vi "oscRead.vi"(0 "input cluster":T2, 1 "error in":errorcluster caption="Error in" {"code" format="%.0x"}) -> (2 "appended array":T1(array[cluster]), 3 "Output String":string, 4 "error out (no error)":errorcluster)   [LabVIEW 2011]
uses:
  Server_Globals.vi
  <instrlib>/niScope/Acquire/Fetch/niScope Multi Fetch Binary 8.vi
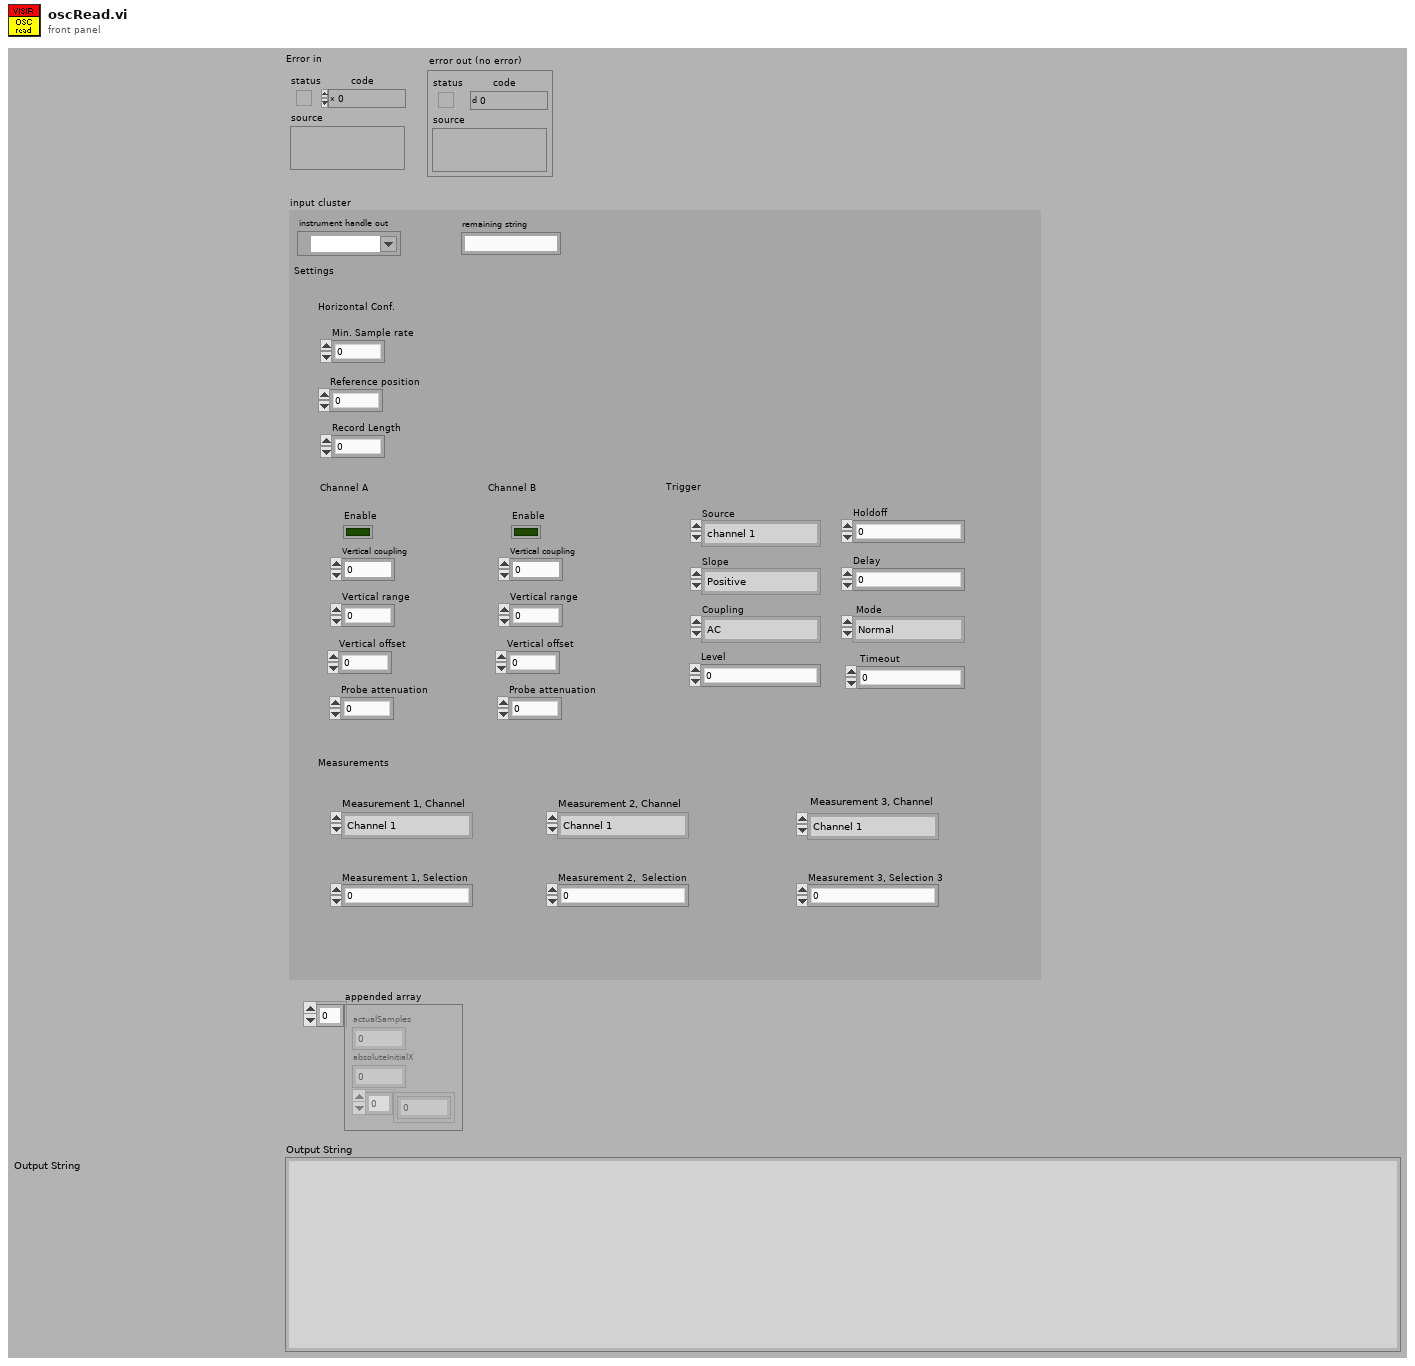
[diagram p1: front panel]
types:
  T1 = cluster{"actualSamples":i32, "absoluteInitialX":dbl, dbl[]}[]
  T2 = cluster{"instrument handle out":refnum<k15>, "remaining string":string, "Settings":cluster{"Horizontal Conf.":cluster{"Min. Sample rate":dbl, "Reference position":dbl, "Record Length":i16}, "Channel A":cluster{"Enable":bool, "Vertical coupling":dbl, "Vertical range":dbl, "Vertical offset":dbl, "Probe attenuation":dbl}, "Channel B":cluster{"Enable":bool, "Vertical coupling":dbl, "Vertical range":dbl, "Vertical offset":dbl, "Probe attenuation":dbl}, "Trigger":cluster{"Source":enum8{"channel 1", "channel 2", "Imediate", "External trigger"}, "Slope":enum8{"Positive", "Negative"}, "Coupling":enum8{"AC", "DC"}, "Level":dbl, "Holdoff":dbl, "Delay":dbl, " Timeout":dbl, " Mode":enum8{"Normal", "Auto", "Auto Level", ""}}, "Measurements":cluster{"Measurement 1, Channel":enum8{"Channel 1", "Channel 2", "Channel 3", "Channel 4"}, "Measurement 1, Selection":dbl, "Measurement 2, Channel":enum8{"Channel 1", "Channel 2", "Channel 3", "Channel 4"}, "Measurement 2,  Selection":dbl, "Measurement 3, Channel":enum8{"Channel 1", "Channel 2", "Channel 3", "Channel 4"}, "Measurement 3, Selection 3":dbl}}}
  T3 = cluster{"I/O Settings":u64[], "Instrument Handle":cluster{"5402":refnum<k15>, " 5112":refnum<k15>, "4072":refnum<k15>, "USB":refnum<visa-resource-name>, "4110":refnum<k15>}, "Logfile":refnum<file>, "Log Level":i8, "Clear":i32[], "OS Set":cluster{"instrument handle out":refnum<k15>, "remaining string":string, "Settings":cluster{"Horizontal Conf.":cluster{"Min. Sample rate":dbl, "Reference position":dbl, "Record Length":i16}, "Channel A":cluster{"Enable":bool, "Vertical coupling":dbl, "Vertical range":dbl, "Vertical offset":dbl, "Probe attenuation":dbl}, "Channel B":cluster{"Enable":bool, "Vertical coupling":dbl, "Vertical range":dbl, "Vertical offset":dbl, "Probe attenuation":dbl}, "Trigger":cluster{"Source":enum8{"channel 1", "channel 2", "Imediate", "External trigger"}, "Slope":enum8{"Positive", "Negative"}, "Coupling":enum8{"AC", "DC"}, "Level":dbl, "Holdoff":dbl, "Delay":dbl, " Timeout":dbl, " Mode":enum8{"Normal", "Auto", "Auto Level"}}, "Measurements":cluster{"Measurement 1, Channel":enum8{"Channel 1", "Channel 2", "Channel 3", "Channel 4"}, "Measurement 1, Selection":u16, "Measurement 2, Channel":enum8{"Channel 1", "Channel 2", "Channel 3", "Channel 4"}, "Measurement 2,  Selection":u16, "Measurement 3, Channel":enum8{"Channel 1", "Channel 2", "Channel 3", "Channel 4"}, "Measurement 3, Selection 3":u16}}}, "DC Power Supply":cluster{"0":refnum<k15>, "1":refnum<k15>, "2":refnum<k15>, "3":refnum<k15>, "4":refnum<k15>}, "USB Interface":cluster{"0":refnum<visa-resource-name>, "1":refnum<visa-resource-name>, "2":refnum<visa-resource-name>, "3":refnum<visa-resource-name>, "4":refnum<visa-resource-name>}, "Function Generator":cluster{"0":refnum<k15>, "1":refnum<k15>, "2":refnum<k15>, "3":refnum<k15>, "4":refnum<k15>}, "Digital Multimeter":cluster{"0":refnum<k15>, "1":refnum<k15>, "2":refnum<k15>, "3":refnum<k15>, "4":refnum<k15>}, "Digital Osciliscope":cluster{"0":refnum<k15>, "1":refnum<k15>, "2":refnum<k15>, "3":refnum<k15>, "4":refnum<k15>}, "To M Server":string, "Adres":string[][], "Matrix version":string, "MD5":string, "Digital Multimeter Card 2":cluster{"0":string, "1":string, "2":string, "3":string, "4":string}}
  T4 = cluster{"0":refnum<k15>, "1":refnum<k15>, "2":refnum<k15>, "3":refnum<k15>, "4":refnum<k15>}
  T5 = cluster{"Measurement 1, Channel":enum8{"Channel 1", "Channel 2", "Channel 3", "Channel 4"}, "Measurement 1, Selection":dbl, "Measurement 2, Channel":enum8{"Channel 1", "Channel 2", "Channel 3", "Channel 4"}, "Measurement 2,  Selection":dbl, "Measurement 3, Channel":enum8{"Channel 1", "Channel 2", "Channel 3", "Channel 4"}, "Measurement 3, Selection 3":dbl}
  T6 = cluster{"actualSamples":i32, "absoluteInitialX":dbl, "relativeInitialX":dbl, "xIncrement":dbl, "offset":dbl, "gain":dbl, "reserved1":dbl, "reserved2":dbl}[]
  T7 = cluster{"Vertical Coupling":i32, "Vertical Coupling":i32}
  T8 = cluster{cluster{"Enable":bool, "Enable":bool}, cluster{"Vertical Coupling":i32, "Vertical Coupling":i32}}
  T9 = cluster{" result ":dbl, " result  2":dbl, " result  3":dbl}
  T10 = cluster{"actualSamples":i32, "absoluteInitialX":dbl, "relativeInitialX":dbl, "xIncrement":dbl, "offset":dbl, "gain":dbl, "reserved1":dbl, "reserved2":dbl}
  T11 = cluster{"actualSamples":i32, "absoluteInitialX":dbl, dbl[]}
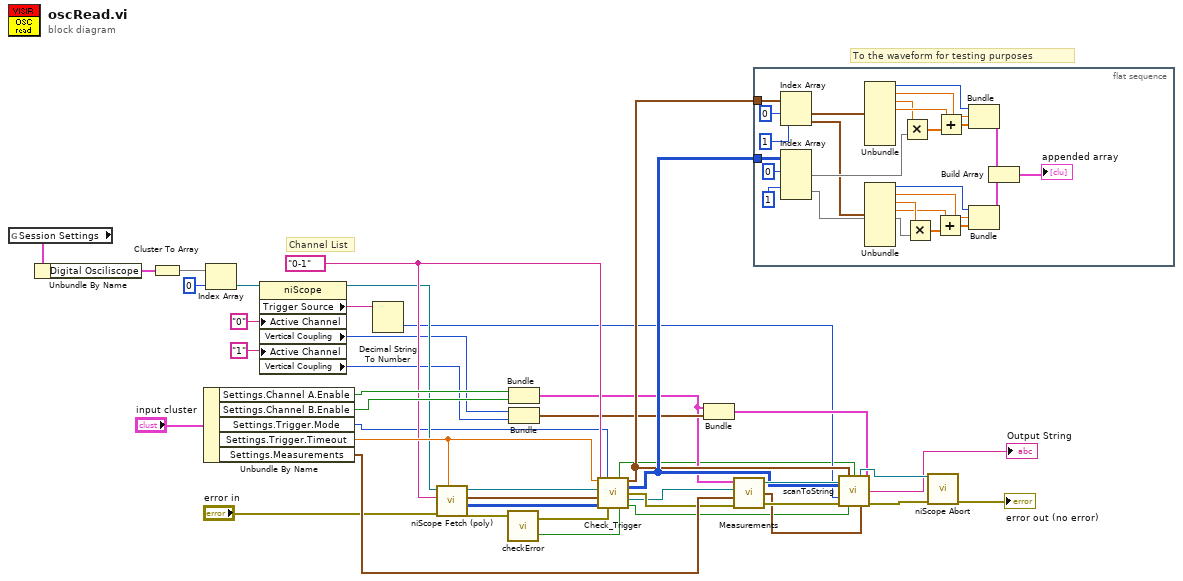
[diagram p0: block diagram]
diagram:
  w20 = "0-1" ("channelList")
  # "Channel List"
  # "To the waveform for testing purposes"
  n1 = global read "Server_Globals.vi" "Session Settings"() -> (w6:T3)
  n2 = Unbundle By Name(w6) -> ("Digital Osciliscope"=w5:T4)
  n3 = Cluster To Array(cluster=w5) -> (array=w4:refnum<k15>[])
  n4 = Unbundle By Name("input cluster") -> ("Settings.Channel A.Enable"=w22:bool, "Settings.Channel B.Enable"=w21:bool, "Settings.Trigger.Mode"=w9:enum8{"Normal", "Auto", "Auto Level", ""}, "Settings.Trigger.Timeout"=w31:dbl, "Settings.Measurements"=w35:T5)
  n5 = Index Array(array=w4, index=0) -> (element=w2:refnum<k15>)
  n6 = property class="niScope"(reference=w2, "Active Channel"="0", "Active Channel"="1") -> (reference out=w14:refnum<k15>, "Trigger Source"=w8:string, "Vertical Coupling"=w11:i32, "Vertical Coupling"=w10:i32)  [unwired: 1 in, 1 out]
  n7 = Decimal String To Number(string=w8) -> (number=w7:i32)  [unwired: 2 in, 1 out]
  n8 = call-poly <instrlib>:"niScope Fetch (poly).vi"("timeout"=w31, "error in"="error in", "channels"=w20, "instrument handle"=w14) -> ("error out"=w40:errorcluster, "wfm"=w29:i8[][], "wfm info"=w41:T6, "instrument handle out"=w30:refnum<k15>)  [unwired: 4 in]
  n9 = call "checkError.vi"("error in"=w40) -> ("Time out"=w33:bool, "error out"=w28:errorcluster)  [unwired: 1 in]
  n10 = Bundle("Enable"=w22, "Enable"=w21) -> (w18:cluster{"Enable":bool, "Enable":bool})  [unwired: 1 in]
  n11 = Bundle("Vertical Coupling"=w11, "Vertical Coupling"=w10) -> (w19:T7)  [unwired: 1 in]
  n12 = call "Check_Trigger.vi"("Timeout"=w31, "Mode"=w9, "instrument handle In"=w30, "channelList"=w20, "wfm info in"=w41, "wfm In"=w29, "error IN"=w28, "Data could not be fetched"=w33) -> ("Immediate trigged"=w1:bool, "wfm info"=w25:T6, "wfm"=w26:i8[][], "error out"=w32:errorcluster, "instrument handle out"=w27:refnum<k15>, "Time out (False when no trigger is found)"=w16:bool)  [unwired: 2 in]
  n13 = Bundle(w18, w19) -> (w17:T8)  [unwired: 1 in]
  n14 = call "Measurements.vi"("error in"=w32, "Measurements"=w35, "instrument handle"=w27, "Enabled Channels cluster"=w18) -> ("error out"=w36:errorcluster, "Measurement results"=w34:T9, "instrument handle out"=w37:refnum<k15>)
  n15 = flat-sequence {
    tunnel: w25 -> [w45]
    tunnel: w26 -> [w44]
    frame #0 {
      n16 = Index Array(array=w45, index #1=0 ("index"), index #2=1 ("index")) -> (element #1=w49:T10, element #2=w52:T10)
      n17 = Index Array(array=w44, index (row) #1=0 ("index (row)"), index (row) #2=1 ("index (row)")) -> (element #1=w60:i8[], element #2=w66:i8[])  [unwired: 2 in]
      n18 = Unbundle(w49) -> ("actualSamples"=w55:i32, "absoluteInitialX"=w56:dbl, "relativeInitialX"=w61:dbl, "xIncrement"=w63:dbl)  [unwired: 4 out]
      n19 = Unbundle(w52) -> ("actualSamples"=w46:i32, "absoluteInitialX"=w57:dbl, "relativeInitialX"=w62:dbl, "xIncrement"=w47:dbl)  [unwired: 4 out]
      n20 = Multiply(x=w61, y=w60) -> (x*y=w64:dbl[])
      n21 = Multiply(x=w62, y=w66) -> (x*y=w48:dbl[])
      n22 = Add(x=w47, y=w48) -> (x+y=w67:dbl[])
      n23 = Add(x=w63, y=w64) -> (x+y=w65:dbl[])
      n24 = Bundle("actualSamples"=w55, "absoluteInitialX"=w56, w65) -> (w59:T11)  [unwired: 1 in]
      n25 = Bundle("actualSamples"=w46, "absoluteInitialX"=w57, w67) -> (w58:T11)  [unwired: 1 in]
      n26 = Build Array(w59, w58) -> (→"appended array":T1)
    }
  }
  n27 = call "scanToString.vi"("instrument handle"=w37, "wfm info"=w25, "Immediate Trigger Received"=w1, "Channels and coupling"=w17, "wfm"=w26, "Triger Source"=w7, "error in"=w36, "Trigger Received"=w16, "Measurements"=w34) -> ("instrument handle out"=w39:refnum<k15>, "Response String"=→"Output String":string, "error out"=w38:errorcluster)  [unwired: 4 in]
  n28 = call <instrlib>:"niScope Abort.vi"("instrument handle"=w39, "error in"=w38) -> ("error out"=→"error out (no error)":errorcluster)  [unwired: 12 in, 1 out]
